vi "gyro-pll-V3.vi"() -> ()   [LabVIEW 2018]
uses:
  lorentzian.ctl
  circle corners.ctl
  pid -- parameters.ctl
  <vilib>/event_ctls.llb/eventvkey.ctl
  show-win- control.ctl
  server talk-to-back pair.ctl
  server talkback message type.ctl
  server talkto message type.ctl
  agregator -- action.ctl
  interpolation state - real.ctl
  pll internal user event action.ctl
  publisher action.ctl
  four-corner circle transformation.ctl
  cursor action.ctl
  Q -- check range -- i -- real.vi
  linear interpolation - real.vi
  draw a circle.vi
  linear interpolation iiii- complex.vi
  <vilib>/Analysis/baseanly.llb/A x B.vi
  <vilib>/Analysis/baseanly.llb/Complex A x B.vi
  line -- complex.vi
  Q -- check range -- i -- integer.vi
  generate linear region.vi
  Q - not nan -- real.vi
  Q - not nan -- integer.vi
  <vilib>/Analysis/Matrix/Numeric/Conversions/Array To Matrix.vi
  <vilib>/Analysis/Matrix/Numeric/Conversions/Array To Matrix - RA2.vi
  <vilib>/Analysis/baseanly.llb/Inverse Matrix.vi
  <vilib>/Analysis/baseanly.llb/Real Inverse Matrix.vi
panel:
  in  "(*) sweeper server":bool=TRUE
  in  "(*) pll":bool
  in  "exit!":bool
  in  "(*) sourcer":bool
  in  "(*) fitter":bool
  in  "(*) sweeper":bool=TRUE
  in  "all 3":T1(tab)
  in  "reset lor! :q":bool
  in  "Tab Control":enum32{"PID", "hist", "params"}(tab)=enum."params"
  in  "PID parameters :{}[];'":T2={"I (sec)"=0.004634123928756344, "P (sec)"=0.008980860327047186} {"P (sec)" scale=0.01..10.0; "I (sec)" scale=0.01..10.0}
  out "Plot: complex- hist":cluster{dbl[], dbl[]}[](graph)=[{array[1000 elements], array[1000 elements]}, {[7.190597353205284e-06, 7.172141018125027e-06, 7.116804391567491e-06, 7.024684552779172e-06, 6.895943111259833e-06, 6.7308059232445354e-06, 6.529562695475053e-06, 6.292566476955803e-06, 6.020233039585921e-06, 5.713040148754082e-06, 5.371526725175644e-06, 4.996291899442611e-06, 4.5879939609449636e-06, 4.147349203007406e-06, 3.6751306662674513e-06, 3.1721667824994774e-06, 2.6393399212638878e-06, 2.0775848419310813e-06, 1.4878870537958579e-06, 8.712810871592677e-07, 2.2884867841089993e-07, -4.382831277042918e-07, -1.1289439553054788e-06, -1.8419221506129192e-06, -2.575966907600425e-06, -3.329790462334158e-06, -4.102070352148148e-06, -4.891451735693187e-06, -5.696549769788949e-06, -6.515952038909475e-06, -7.348221033039968e-06, -8.191896669557811e-06, -9.045498854713654e-06, -9.907530080218758e-06, -1.0776478050383408e-05, -1.1650818335197432e-05, -1.252901704469844e-05, -1.3409533519936043e-05, -1.4290823035811157e-05, -1.5171339511048758e-05, -1.6049538220549768e-05, -1.692387850536379e-05, -1.7792826475528438e-05, -1.8654857701033543e-05, -1.950845988618939e-05, -2.035213552270723e-05, -2.1184404516837726e-05, -2.200380678595825e-05, -2.2808904820054008e-05, -2.3598286203599055e-05, -2.4370566093413044e-05, -2.5124389648146775e-05, -2.5858434405134282e-05, -2.6571412600441725e-05, -2.7262073428042906e-05, -2.79292052341581e-05, -2.8571637642906468e-05, -2.918824360954306e-05, -2.9777941397678286e-05, -3.0339696477011096e-05, -3.087252333824668e-05, -3.137548722201465e-05, -3.184770575875461e-05, -3.228835051669217e-05, -3.269664845518981e-05, -3.3071883280922845e-05, -3.341339670450129e-05, -3.372058959533313e-05, -3.399292303270301e-05, -3.4229919251222255e-05, -3.4431162478991744e-05, -3.4596299667007035e-05, -3.472504110852638e-05, -3.4817160947314696e-05, -3.4872497573872235e-05, -3.489095390895249e-05, -3.4872497573872235e-05, -3.4817160947314696e-05, -3.472504110852638e-05, -3.459629966700704e-05, -3.4431162478991744e-05, -3.422991925122226e-05, -3.3992923032703014e-05, -3.372058959533313e-05, -3.341339670450129e-05, -3.307188328092285e-05, -3.269664845518982e-05, -3.2288350516692175e-05, -3.1847705758754615e-05, -3.137548722201466e-05, -3.087252333824669e-05, -3.0339696477011103e-05, -2.9777941397678293e-05, -2.9188243609543066e-05, -2.8571637642906474e-05, -2.7929205234158112e-05, -2.726207342804292e-05, -2.6571412600441735e-05, -2.5858434405134296e-05, -2.512438964814679e-05, -2.4370566093413057e-05, -2.3598286203599066e-05, -2.280890482005402e-05, -2.200380678595826e-05, -2.1184404516837737e-05, -2.035213552270724e-05, -1.9508459886189396e-05, -1.865485770103357e-05, -1.7792826475528462e-05, -1.6923878505363813e-05, -1.6049538220549788e-05, -1.5171339511048779e-05, -1.4290823035811176e-05, -1.3409533519936056e-05, -1.2529017044698455e-05, -1.1650818335197446e-05, -1.0776478050383421e-05, -9.907530080218769e-06, -9.045498854713664e-06, -8.19189666955782e-06, -7.348221033039972e-06, -6.515952038909498e-06, -5.69654976978897e-06, -4.891451735693207e-06, -4.102070352148165e-06, -3.3297904623341733e-06, -2.575966907600442e-06, -1.8419221506129327e-06, -1.1289439553054907e-06, -4.3828312770430365e-07, 2.2884867841089146e-07, 8.712810871592576e-07, 1.4878870537958511e-06, 2.0775848419310745e-06, 2.6393399212638844e-06, 3.172166782499474e-06, 3.6751306662674378e-06, 4.147349203007396e-06, 4.587993960944957e-06, 4.996291899442601e-06, 5.371526725175637e-06, 5.713040148754075e-06, 6.020233039585914e-06, 6.292566476955799e-06, 6.52956269547505e-06, 6.7308059232445354e-06, 6.89594311125983e-06, 7.024684552779168e-06, 7.116804391567491e-06, 7.172141018125027e-06], [0.0002113633008955132, 0.00021224439713003404, 0.00021312394762236102, 0.00021400040934205735, 0.00021487224467744295, 0.00021573792413308792, 0.00021659592901306725, 0.0002174447540852694, 0.00021828291022208502, 0.0002191089270128428, 0.00021992135534340933, 0.00022071876993842783, 0.00022149977186173528, 0.00022226299097057205, 0.00022300708831927754, 0.00022373075850825623, 0.00022443273197409182, 0.00022511177721679307, 0.00022576670296026313, 0.00022639636024220273, 0.00022699964442978034, 0.0002275754971575336, 0.000228122908184102, 0.00022864091716453335, 0.0002291286153350554, 0.0002295851471073561, 0.00023000971156957625, 0.00023040156389138116, 0.0002307600166306461, 0.00023108444093946333, 0.00023137426766735506, 0.00023162898835975677, 0.0002318481561500193, 0.00023203138654336486, 0.0002321783580914214, 0.00023228881295615236, 0.00023236255736219216, 0.00023239946193679412, 0.00023239946193679412, 0.00023236255736219216, 0.00023228881295615236, 0.0002321783580914214, 0.00023203138654336486, 0.0002318481561500193, 0.00023162898835975677, 0.00023137426766735506, 0.00023108444093946333, 0.00023076001663064613, 0.00023040156389138116, 0.00023000971156957625, 0.0002295851471073561, 0.0002291286153350554, 0.00022864091716453335, 0.000228122908184102, 0.0002275754971575336, 0.00022699964442978034, 0.00022639636024220273, 0.00022576670296026315, 0.00022511177721679307, 0.00022443273197409182, 0.00022373075850825623, 0.00022300708831927757, 0.00022226299097057205, 0.0002214997718617353, 0.00022071876993842783, 0.00021992135534340933, 0.0002191089270128428, 0.00021828291022208502, 0.0002174447540852694, 0.00021659592901306725, 0.00021573792413308792, 0.00021487224467744295, 0.00021400040934205735, 0.00021312394762236102, 0.00021224439713003404, 0.0002113633008955132, 0.00021048220466099237, 0.0002096026541686654, 0.0002087261924489691, 0.0002078543571135835, 0.0002069886776579385, 0.00020613067277795916, 0.00020528184770575705, 0.00020444369156894142, 0.00020361767477818362, 0.00020280524644761708, 0.0002020078318525986, 0.00020122682992929113, 0.0002004636108204544, 0.00019971951347174887, 0.00019899584328277018, 0.0001982938698169346, 0.00019761482457423337, 0.0001969598988307633, 0.00019633024154882368, 0.00019572695736124607, 0.0001951511046334928, 0.00019460369360692445, 0.00019408568462649307, 0.00019359798645597102, 0.00019314145468367035, 0.0001927168902214502, 0.00019232503789964525, 0.0001919665851603803, 0.00019164216085156309, 0.00019135233412367135, 0.00019109761343126964, 0.0001908784456410071, 0.00019069521524766155, 0.000190548243699605, 0.00019043778883487406, 0.00019036404442883425, 0.0001903271398542323, 0.0001903271398542323, 0.00019036404442883425, 0.00019043778883487406, 0.000190548243699605, 0.00019069521524766155, 0.0001908784456410071, 0.00019109761343126964, 0.00019135233412367135, 0.00019164216085156306, 0.00019196658516038029, 0.00019232503789964523, 0.00019271689022145016, 0.00019314145468367033, 0.000193597986455971, 0.00019408568462649307, 0.00019460369360692443, 0.0001951511046334928, 0.00019572695736124607, 0.00019633024154882368, 0.00019695989883076326, 0.00019761482457423334, 0.0001982938698169346, 0.00019899584328277018, 0.00019971951347174885, 0.00020046361082045436, 0.0002012268299292911, 0.00020200783185259858, 0.00020280524644761705, 0.0002036176747781836, 0.0002044436915689414, 0.00020528184770575702, 0.00020613067277795916, 0.0002069886776579385, 0.00020785435711358346, 0.00020872619244896907, 0.00020960265416866537, 0.00021048220466099237]}, {[7.168586400274939e-06, 5.066709932460086e-06, 2.964833464645231e-06, 8.629569968303764e-07, -1.2389194709844774e-06, -3.340795938799331e-06, -5.442672406614187e-06, -7.54454887442904e-06, -9.646425342243894e-06, -1.174830181005875e-05, -1.3850178277873602e-05, -1.5952054745688457e-05, -1.8053931213503313e-05, -2.0155807681318165e-05, -2.225768414913302e-05, -2.4359560616947872e-05, -2.6461437084762728e-05, -2.8563313552577583e-05, -3.066519002039244e-05, -3.276706648820729e-05], [0.00021232547061132137, 0.00021222925363974056, 0.00021213303666815973, 0.00021203681969657892, 0.0002119406027249981, 0.0002118443857534173, 0.00021174816878183648, 0.00021165195181025565, 0.00021155573483867484, 0.000211459517867094, 0.0002113633008955132, 0.0002112670839239324, 0.00021117086695235157, 0.00021107464998077076, 0.00021097843300918993, 0.00021088221603760913, 0.00021078599906602832, 0.0002106897820944475, 0.00021059356512286668, 0.00021049734815128585]}, {[-1.288800856206544e-05, -1.2984225533646258e-05, -1.3080442505227073e-05, -1.317665947680789e-05, -1.3272876448388706e-05, -1.3369093419969523e-05, -1.3465310391550338e-05, -1.3561527363131155e-05, -1.365774433471197e-05, -1.3753961306292788e-05, -1.3850178277873605e-05, -1.394639524945442e-05, -1.4042612221035236e-05, -1.4138829192616053e-05, -1.423504616419687e-05, -1.4331263135777686e-05, -1.4427480107358503e-05, -1.4523697078939318e-05, -1.4619914050520135e-05, -1.471613102210095e-05], [0.00019034453621736468, 0.00019244641268517952, 0.0001945482891529944, 0.00019665016562080923, 0.0001987520420886241, 0.00020085391855643894, 0.00020295579502425378, 0.00020505767149206865, 0.0002071595479598835, 0.00020926142442769836, 0.0002113633008955132, 0.00021346517736332805, 0.00021556705383114292, 0.00021766893029895776, 0.00021977080676677263, 0.00022187268323458747, 0.0002239745597024023, 0.00022607643617021718, 0.00022817831263803202, 0.0002302801891058469]}, {[9.092925831891258e-06, 8.900491888729626e-06, 8.708057945567993e-06, 8.515624002406362e-06, 8.32319005924473e-06, 8.130756116083097e-06, 7.938322172921465e-06, 7.745888229759832e-06, 7.5534542865982e-06, 7.361020343436568e-06, 7.168586400274936e-06, 6.976152457113303e-06, 6.783718513951671e-06, 6.591284570790038e-06, 6.3988506276284065e-06, 6.206416684466774e-06, 6.013982741305142e-06, 5.82154879814351e-06, 5.629114854981877e-06, 5.4366809118202445e-06], [0.0001702879412550243, 0.00017449169419065402, 0.00017869544712628373, 0.00018289920006191342, 0.00018710295299754313, 0.00019130670593317284, 0.00019551045886880255, 0.00019971421180443226, 0.00020391796474006197, 0.00020812171767569168, 0.00021232547061132137, 0.00021652922354695108, 0.0002207329764825808, 0.0002249367294182105, 0.0002291404823538402, 0.0002333442352894699, 0.00023754798822509963, 0.00024175174116072932, 0.00024595549409635905, 0.00025015924703198874]}, {[-1.97103396318906e-05, -1.91243234964889e-05, -1.8538307361087202e-05, -1.79522912256855e-05, -1.73662750902838e-05, -1.6780258954882103e-05, -1.6194242819480402e-05, -1.5608226684078704e-05, -1.5022210548677003e-05, -1.4436194413275303e-05, -1.3850178277873603e-05, -1.3264162142471904e-05, -1.2678146007070203e-05, -1.2092129871668504e-05, -1.1506113736266805e-05, -1.0920097600865104e-05, -1.0334081465463405e-05, -9.748065330061706e-06, -9.162049194660005e-06, -8.576033059258306e-06], [0.00023375398508080204, 0.00023151491666227315, 0.00022927584824374426, 0.0002270367798252154, 0.0002247977114066865, 0.00022255864298815762, 0.00022031957456962873, 0.00021808050615109985, 0.00021584143773257098, 0.0002136023693140421, 0.0002113633008955132, 0.00020912423247698432, 0.00020688516405845543, 0.00020464609563992657, 0.00020240702722139768, 0.0002001679588028688, 0.0001979288903843399, 0.00019568982196581104, 0.00019345075354728215, 0.00019121168512875326]}]
  in  "dt (sec)":dbl=0.001 format="%#_10f"
  in  "plot hist time (sec)":dbl=1.0 format="%#_10f"
  out "G (Hz)":dbl=6.817921124952451 format="%#.4f"
  in  "reset freq! :r":bool
  out "Plot: complex plane":cluster{dbl[], dbl[]}[](graph)=[{[7.190597353205284e-06, 7.172141018125027e-06, 7.116804391567491e-06, 7.024684552779172e-06, 6.895943111259833e-06, 6.7308059232445354e-06, 6.529562695475053e-06, 6.292566476955803e-06, 6.020233039585921e-06, 5.713040148754082e-06, 5.371526725175644e-06, 4.996291899442611e-06, 4.5879939609449636e-06, 4.147349203007406e-06, 3.6751306662674513e-06, 3.1721667824994774e-06, 2.6393399212638878e-06, 2.0775848419310813e-06, 1.4878870537958579e-06, 8.712810871592677e-07, 2.2884867841089993e-07, -4.382831277042918e-07, -1.1289439553054788e-06, -1.8419221506129192e-06, -2.575966907600425e-06, -3.329790462334158e-06, -4.102070352148148e-06, -4.891451735693187e-06, -5.696549769788949e-06, -6.515952038909475e-06, -7.348221033039968e-06, -8.191896669557811e-06, -9.045498854713654e-06, -9.907530080218758e-06, -1.0776478050383408e-05, -1.1650818335197432e-05, -1.252901704469844e-05, -1.3409533519936043e-05, -1.4290823035811157e-05, -1.5171339511048758e-05, -1.6049538220549768e-05, -1.692387850536379e-05, -1.7792826475528438e-05, -1.8654857701033543e-05, -1.950845988618939e-05, -2.035213552270723e-05, -2.1184404516837726e-05, -2.200380678595825e-05, -2.2808904820054008e-05, -2.3598286203599055e-05, -2.4370566093413044e-05, -2.5124389648146775e-05, -2.5858434405134282e-05, -2.6571412600441725e-05, -2.7262073428042906e-05, -2.79292052341581e-05, -2.8571637642906468e-05, -2.918824360954306e-05, -2.9777941397678286e-05, -3.0339696477011096e-05, -3.087252333824668e-05, -3.137548722201465e-05, -3.184770575875461e-05, -3.228835051669217e-05, -3.269664845518981e-05, -3.3071883280922845e-05, -3.341339670450129e-05, -3.372058959533313e-05, -3.399292303270301e-05, -3.4229919251222255e-05, -3.4431162478991744e-05, -3.4596299667007035e-05, -3.472504110852638e-05, -3.4817160947314696e-05, -3.4872497573872235e-05, -3.489095390895249e-05, -3.4872497573872235e-05, -3.4817160947314696e-05, -3.472504110852638e-05, -3.459629966700704e-05, -3.4431162478991744e-05, -3.422991925122226e-05, -3.3992923032703014e-05, -3.372058959533313e-05, -3.341339670450129e-05, -3.307188328092285e-05, -3.269664845518982e-05, -3.2288350516692175e-05, -3.1847705758754615e-05, -3.137548722201466e-05, -3.087252333824669e-05, -3.0339696477011103e-05, -2.9777941397678293e-05, -2.9188243609543066e-05, -2.8571637642906474e-05, -2.7929205234158112e-05, -2.726207342804292e-05, -2.6571412600441735e-05, -2.5858434405134296e-05, -2.512438964814679e-05, -2.4370566093413057e-05, -2.3598286203599066e-05, -2.280890482005402e-05, -2.200380678595826e-05, -2.1184404516837737e-05, -2.035213552270724e-05, -1.9508459886189396e-05, -1.865485770103357e-05, -1.7792826475528462e-05, -1.6923878505363813e-05, -1.6049538220549788e-05, -1.5171339511048779e-05, -1.4290823035811176e-05, -1.3409533519936056e-05, -1.2529017044698455e-05, -1.1650818335197446e-05, -1.0776478050383421e-05, -9.907530080218769e-06, -9.045498854713664e-06, -8.19189666955782e-06, -7.348221033039972e-06, -6.515952038909498e-06, -5.69654976978897e-06, -4.891451735693207e-06, -4.102070352148165e-06, -3.3297904623341733e-06, -2.575966907600442e-06, -1.8419221506129327e-06, -1.1289439553054907e-06, -4.3828312770430365e-07, 2.2884867841089146e-07, 8.712810871592576e-07, 1.4878870537958511e-06, 2.0775848419310745e-06, 2.6393399212638844e-06, 3.172166782499474e-06, 3.6751306662674378e-06, 4.147349203007396e-06, 4.587993960944957e-06, 4.996291899442601e-06, 5.371526725175637e-06, 5.713040148754075e-06, 6.020233039585914e-06, 6.292566476955799e-06, 6.52956269547505e-06, 6.7308059232445354e-06, 6.89594311125983e-06, 7.024684552779168e-06, 7.116804391567491e-06, 7.172141018125027e-06], [0.0002113633008955132, 0.00021224439713003404, 0.00021312394762236102, 0.00021400040934205735, 0.00021487224467744295, 0.00021573792413308792, 0.00021659592901306725, 0.0002174447540852694, 0.00021828291022208502, 0.0002191089270128428, 0.00021992135534340933, 0.00022071876993842783, 0.00022149977186173528, 0.00022226299097057205, 0.00022300708831927754, 0.00022373075850825623, 0.00022443273197409182, 0.00022511177721679307, 0.00022576670296026313, 0.00022639636024220273, 0.00022699964442978034, 0.0002275754971575336, 0.000228122908184102, 0.00022864091716453335, 0.0002291286153350554, 0.0002295851471073561, 0.00023000971156957625, 0.00023040156389138116, 0.0002307600166306461, 0.00023108444093946333, 0.00023137426766735506, 0.00023162898835975677, 0.0002318481561500193, 0.00023203138654336486, 0.0002321783580914214, 0.00023228881295615236, 0.00023236255736219216, 0.00023239946193679412, 0.00023239946193679412, 0.00023236255736219216, 0.00023228881295615236, 0.0002321783580914214, 0.00023203138654336486, 0.0002318481561500193, 0.00023162898835975677, 0.00023137426766735506, 0.00023108444093946333, 0.00023076001663064613, 0.00023040156389138116, 0.00023000971156957625, 0.0002295851471073561, 0.0002291286153350554, 0.00022864091716453335, 0.000228122908184102, 0.0002275754971575336, 0.00022699964442978034, 0.00022639636024220273, 0.00022576670296026315, 0.00022511177721679307, 0.00022443273197409182, 0.00022373075850825623, 0.00022300708831927757, 0.00022226299097057205, 0.0002214997718617353, 0.00022071876993842783, 0.00021992135534340933, 0.0002191089270128428, 0.00021828291022208502, 0.0002174447540852694, 0.00021659592901306725, 0.00021573792413308792, 0.00021487224467744295, 0.00021400040934205735, 0.00021312394762236102, 0.00021224439713003404, 0.0002113633008955132, 0.00021048220466099237, 0.0002096026541686654, 0.0002087261924489691, 0.0002078543571135835, 0.0002069886776579385, 0.00020613067277795916, 0.00020528184770575705, 0.00020444369156894142, 0.00020361767477818362, 0.00020280524644761708, 0.0002020078318525986, 0.00020122682992929113, 0.0002004636108204544, 0.00019971951347174887, 0.00019899584328277018, 0.0001982938698169346, 0.00019761482457423337, 0.0001969598988307633, 0.00019633024154882368, 0.00019572695736124607, 0.0001951511046334928, 0.00019460369360692445, 0.00019408568462649307, 0.00019359798645597102, 0.00019314145468367035, 0.0001927168902214502, 0.00019232503789964525, 0.0001919665851603803, 0.00019164216085156309, 0.00019135233412367135, 0.00019109761343126964, 0.0001908784456410071, 0.00019069521524766155, 0.000190548243699605, 0.00019043778883487406, 0.00019036404442883425, 0.0001903271398542323, 0.0001903271398542323, 0.00019036404442883425, 0.00019043778883487406, 0.000190548243699605, 0.00019069521524766155, 0.0001908784456410071, 0.00019109761343126964, 0.00019135233412367135, 0.00019164216085156306, 0.00019196658516038029, 0.00019232503789964523, 0.00019271689022145016, 0.00019314145468367033, 0.000193597986455971, 0.00019408568462649307, 0.00019460369360692443, 0.0001951511046334928, 0.00019572695736124607, 0.00019633024154882368, 0.00019695989883076326, 0.00019761482457423334, 0.0001982938698169346, 0.00019899584328277018, 0.00019971951347174885, 0.00020046361082045436, 0.0002012268299292911, 0.00020200783185259858, 0.00020280524644761705, 0.0002036176747781836, 0.0002044436915689414, 0.00020528184770575702, 0.00020613067277795916, 0.0002069886776579385, 0.00020785435711358346, 0.00020872619244896907, 0.00020960265416866537, 0.00021048220466099237]}, {[7.168586400274939e-06, 5.066709932460086e-06, 2.964833464645231e-06, 8.629569968303764e-07, -1.2389194709844774e-06, -3.340795938799331e-06, -5.442672406614187e-06, -7.54454887442904e-06, -9.646425342243894e-06, -1.174830181005875e-05, -1.3850178277873602e-05, -1.5952054745688457e-05, -1.8053931213503313e-05, -2.0155807681318165e-05, -2.225768414913302e-05, -2.4359560616947872e-05, -2.6461437084762728e-05, -2.8563313552577583e-05, -3.066519002039244e-05, -3.276706648820729e-05], [0.00021232547061132137, 0.00021222925363974056, 0.00021213303666815973, 0.00021203681969657892, 0.0002119406027249981, 0.0002118443857534173, 0.00021174816878183648, 0.00021165195181025565, 0.00021155573483867484, 0.000211459517867094, 0.0002113633008955132, 0.0002112670839239324, 0.00021117086695235157, 0.00021107464998077076, 0.00021097843300918993, 0.00021088221603760913, 0.00021078599906602832, 0.0002106897820944475, 0.00021059356512286668, 0.00021049734815128585]}, {[-1.288800856206544e-05, -1.2984225533646258e-05, -1.3080442505227073e-05, -1.317665947680789e-05, -1.3272876448388706e-05, -1.3369093419969523e-05, -1.3465310391550338e-05, -1.3561527363131155e-05, -1.365774433471197e-05, -1.3753961306292788e-05, -1.3850178277873605e-05, -1.394639524945442e-05, -1.4042612221035236e-05, -1.4138829192616053e-05, -1.423504616419687e-05, -1.4331263135777686e-05, -1.4427480107358503e-05, -1.4523697078939318e-05, -1.4619914050520135e-05, -1.471613102210095e-05], [0.00019034453621736468, 0.00019244641268517952, 0.0001945482891529944, 0.00019665016562080923, 0.0001987520420886241, 0.00020085391855643894, 0.00020295579502425378, 0.00020505767149206865, 0.0002071595479598835, 0.00020926142442769836, 0.0002113633008955132, 0.00021346517736332805, 0.00021556705383114292, 0.00021766893029895776, 0.00021977080676677263, 0.00022187268323458747, 0.0002239745597024023, 0.00022607643617021718, 0.00022817831263803202, 0.0002302801891058469]}, {[9.092925831891258e-06, 8.900491888729626e-06, 8.708057945567993e-06, 8.515624002406362e-06, 8.32319005924473e-06, 8.130756116083097e-06, 7.938322172921465e-06, 7.745888229759832e-06, 7.5534542865982e-06, 7.361020343436568e-06, 7.168586400274936e-06, 6.976152457113303e-06, 6.783718513951671e-06, 6.591284570790038e-06, 6.3988506276284065e-06, 6.206416684466774e-06, 6.013982741305142e-06, 5.82154879814351e-06, 5.629114854981877e-06, 5.4366809118202445e-06], [0.0001702879412550243, 0.00017449169419065402, 0.00017869544712628373, 0.00018289920006191342, 0.00018710295299754313, 0.00019130670593317284, 0.00019551045886880255, 0.00019971421180443226, 0.00020391796474006197, 0.00020812171767569168, 0.00021232547061132137, 0.00021652922354695108, 0.0002207329764825808, 0.0002249367294182105, 0.0002291404823538402, 0.0002333442352894699, 0.00023754798822509963, 0.00024175174116072932, 0.00024595549409635905, 0.00025015924703198874]}]
  in  "lorentzian":T3={"A (VHz)"=0.0007250653088846297, "f (Hz)"=45017.43809779818, "G (Hz)"=34.46000858512321, "phi(rad)"=-1.525051560312372, "Q"=1306.3675821959234, "Norm  Ampl"=nan, "bg (V)"=7.168586400274938e-06+0.00021232547061132137i, "4corners"={"z (-pi/2)"=-1.288800856206544e-05+0.00019034453621736468i, "z(inf)"=7.168586400274938e-06+0.00021232547061132137i, "z (pi/2)"=-1.4812347993681768e-05+0.00023238206557366173i, "z center"=-1.3850178277873603e-05+0.0002113633008955132i, "z(0)"=-3.486894295602214e-05+0.00021040113117970505i, "radius"=2.1040775631078887e-05}} {"bg (V)" format="%#9_9f"; "Q" format="%#9_9f"; "phi(rad)" format="%#9_9f"; "G (Hz)" format="%#9_9f"; "f (Hz)" format="%#9_9f"}
  in  "toggle PLL! :@":bool
  out "f (Hz)":dbl=40017.438097734725 format="%#.11f"
  in  "PLL is ON":bool
  out "VKey":T5
  out "Char":i16=62
  in  "lorentzian -- basic":T3={"A (VHz)"=1.0, "f (Hz)"=1000.0, "G (Hz)"=3.0, "phi(rad)"=0.0, "Q"=300.0, "Norm  Ampl"=nan, "bg (V)"=0.0+0.0i, "4corners"={"z (-pi/2)"=9.277908004825974e-07+0.0007240755403629966i, "z(inf)"=2.6527949823343002e-05+0.0007477540585896028i, "z (pi/2)"=2.8494315967368497e-06+0.0007733542176124632i, "z center"=1.8886111986097237e-06+0.0007487148789877299i, "z(0)"=-2.2750727426123552e-05+0.000749675699385857i, "radius"=2.4658065287076567e-05}} {"bg (V)" format="%#9_9f"; "Q" format="%#9_9f"; "phi(rad)" format="%#9_9f"; "G (Hz)" format="%#9_9f"; "f (Hz)" format="%#9_9f"}
  in  "save lor for later":bool
  in  "reset lorentzian from basic":bool
  out "zi out Im (V)":dbl=-2.55535250615244e-07 format="%#.8f"
  out "zi out Re (V)":dbl=2.3785838016890924e-07 format="%#.8f"
  out "publish message":T6
  out "Stoped?":bool
  out "window":T7={"cen (Hz)"=45496.74569300777, "win (Hz)"=29.962105514646385, "left (Hz)"=45481.76464025045, "right (Hz)"=45511.72674576509}
  in  "lorentzian -- hist":T3={"A (VHz)"=0.0007250653088846297, "f (Hz)"=45017.43809779818, "G (Hz)"=34.46000858512321, "phi(rad)"=-1.525051560312372, "Q"=1306.3675821959234, "Norm  Ampl"=nan, "bg (V)"=7.168586400274938e-06+0.00021232547061132137i, "4corners"={"z (-pi/2)"=-1.288800856206544e-05+0.00019034453621736468i, "z(inf)"=7.168586400274938e-06+0.00021232547061132137i, "z (pi/2)"=-1.4812347993681768e-05+0.00023238206557366173i, "z center"=-1.3850178277873603e-05+0.0002113633008955132i, "z(0)"=-3.486894295602214e-05+0.00021040113117970505i, "radius"=2.1040775631078887e-05}} {"bg (V)" format="%#9_9f"; "Q" format="%#9_9f"; "phi(rad)" format="%#9_9f"; "G (Hz)" format="%#9_9f"; "f (Hz)" format="%#9_9f"}
  out "pll event pair":T8
  out "sweeper server reference":refnum<vi>
  out "pll async reference":refnum<vi>
  out "async fitter":refnum<vi>
  out "async sweeper":refnum<vi>
  out "fitter event pair":T8
  out "sweeper event pair":T8
  out "async sourcer":refnum<vi>
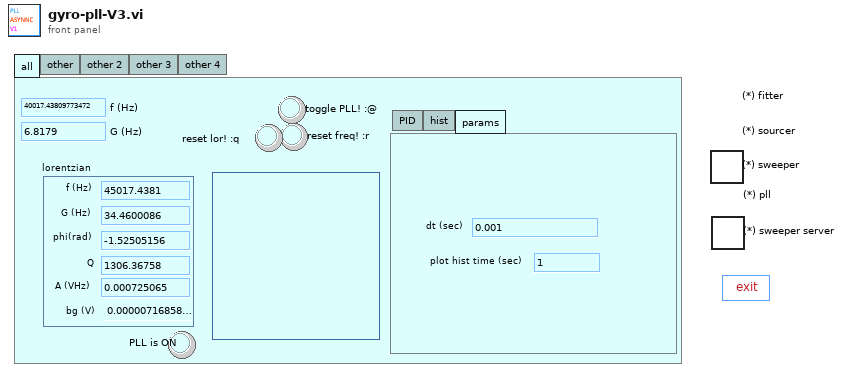
[diagram p1: front panel]
types:
  T1 = enum32{"all", "other", "other 2", "other 3", "other 4"}
  T2 = typedef "pid -- parameters.ctl" = cluster{"I (sec)":dbl, "P (sec)":dbl}
  T3 = typedef "lorentzian.ctl" = cluster{"A (VHz)":dbl, "f (Hz)":dbl, "G (Hz)":dbl, "phi(rad)":dbl, "Q":dbl, "Norm  Ampl":dbl, "bg (V)":cdb, "4corners":T4}
  T4 = typedef "circle corners.ctl" = cluster{"z (-pi/2)":cdb, "z(inf)":cdb, "z (pi/2)":cdb, "z center":cdb, "z(0)":cdb, "radius":dbl}
  T5 = typedef "eventvkey.ctl" = enum16{"ASCII", "Enter", "Return", "Shift", "Ctrl", "Alt", "Cmd", "Opt", "Caps", "NumLock", "Clear", "Break", "Up", "Down", "Left", "Right", "Insert", "Delete", "Home", "End", "PageUp", "PageDown", "Escape", "Help", "Pause", "ScrollLock", "F1", "F2", "F3", "F4", "F5", "F6", "F7", "F8", "F9", "F10", "F11", "F12", "F13", "F14", "F15", "F16", "F17", "F18", "F19", "F20", "F21", "F22", "F23", "F24", "Play", "VolumeUp", "VolumeDown", "Mute", "Two Byte Char"}
  T6 = cluster{"freq (Hz)":dbl, "gamma (Hz)":dbl, "Voltage (V)":cdb}
  T7 = typedef "show-win- control.ctl" = cluster{"cen (Hz)":dbl, "win (Hz)":dbl, "left (Hz)":dbl, "right (Hz)":dbl}
  T8 = typedef "server talk-to-back pair.ctl" = cluster{"talkback event":refnum<user-event>, "talkto event":refnum<user-event>}
  T9 = typedef "server talkback message type.ctl" = cluster{"message":enum16{"new", "void"}}
  T10 = typedef "server talkto message type.ctl" = cluster{"message":enum16{"stop", "start", "update pars", "update request", "new", "launch", "exit", "get", "reset", "pause", "unpause"}}
  T11 = typedef "pll internal user event action.ctl" = enum16{"gear pll async", "start pll async", "stop pll async", "toggle pll async", "gear sweeper", "start sweeper", "stop sweeper", "toggle sweeper", "accept frequency", "reset lorentzian", "accept lorentzian", "update cursors", "pause pll", "unpause pll", "void", "exit", "gear server sweeper", "gear sweeper async", "gear fitter", "gear sourcer"}
  T12 = typedef "interpolation state - real.ctl" = cluster{"requested size":i32, "Array":dbl[], "actual number of elements":i32}
  T13 = typedef "agregator -- action.ctl" = enum16{"append", "interpolate", "empty!", "force", "init", "scale", "read last"}
  T14 = typedef "publisher action.ctl" = enum16{"set", "get", "init", "check"}
  T15 = typedef "cursor action.ctl" = enum16{"range", "read", "write", "check", "zoom out", "smart zoom out", "zoom to aspect ratio 1", "zoom to win", "zoom out 20%", "zoom in 20%", "-empty", "smart zoom out&aspect", "move range left 20%", "move range right 20%", "move range up 20%", "move range down 20%", "zoom to X win", "zoom to Y win", "zoom out X", "zoom out Y", "zoom in X", "zoom in Y", "check plot scale"}
  T16 = typedef "four-corner circle transformation.ctl" = enum16{"z(c) z(inf)", "z(c) z(zero)", "fix phase", "calculate lorentzian", "z(0) z(+-pi/2)", "shift to zcenter", "to  canonical", "get canonical phase", "get4corners", "update lorentzian -- from z0", "fake gamma normal", "fake gamma heat", "calculate complex slope"}
  T17 = typedef "pll talkback data type.ctl" = cluster{"freq (Hz)":dbl, "gamma (Hz)":dbl, "Voltage (V)":cdb, "overlimit ?":bool}
  T18 = typedef "interpolation state - complex.ctl" = cluster{"requested size":i32, "Array":cdb[], "actual number of elements":i32}
  T19 = enum32{"Invalid", "Standard", "Closed", "Hidden", "Minimized", "Maximized"}
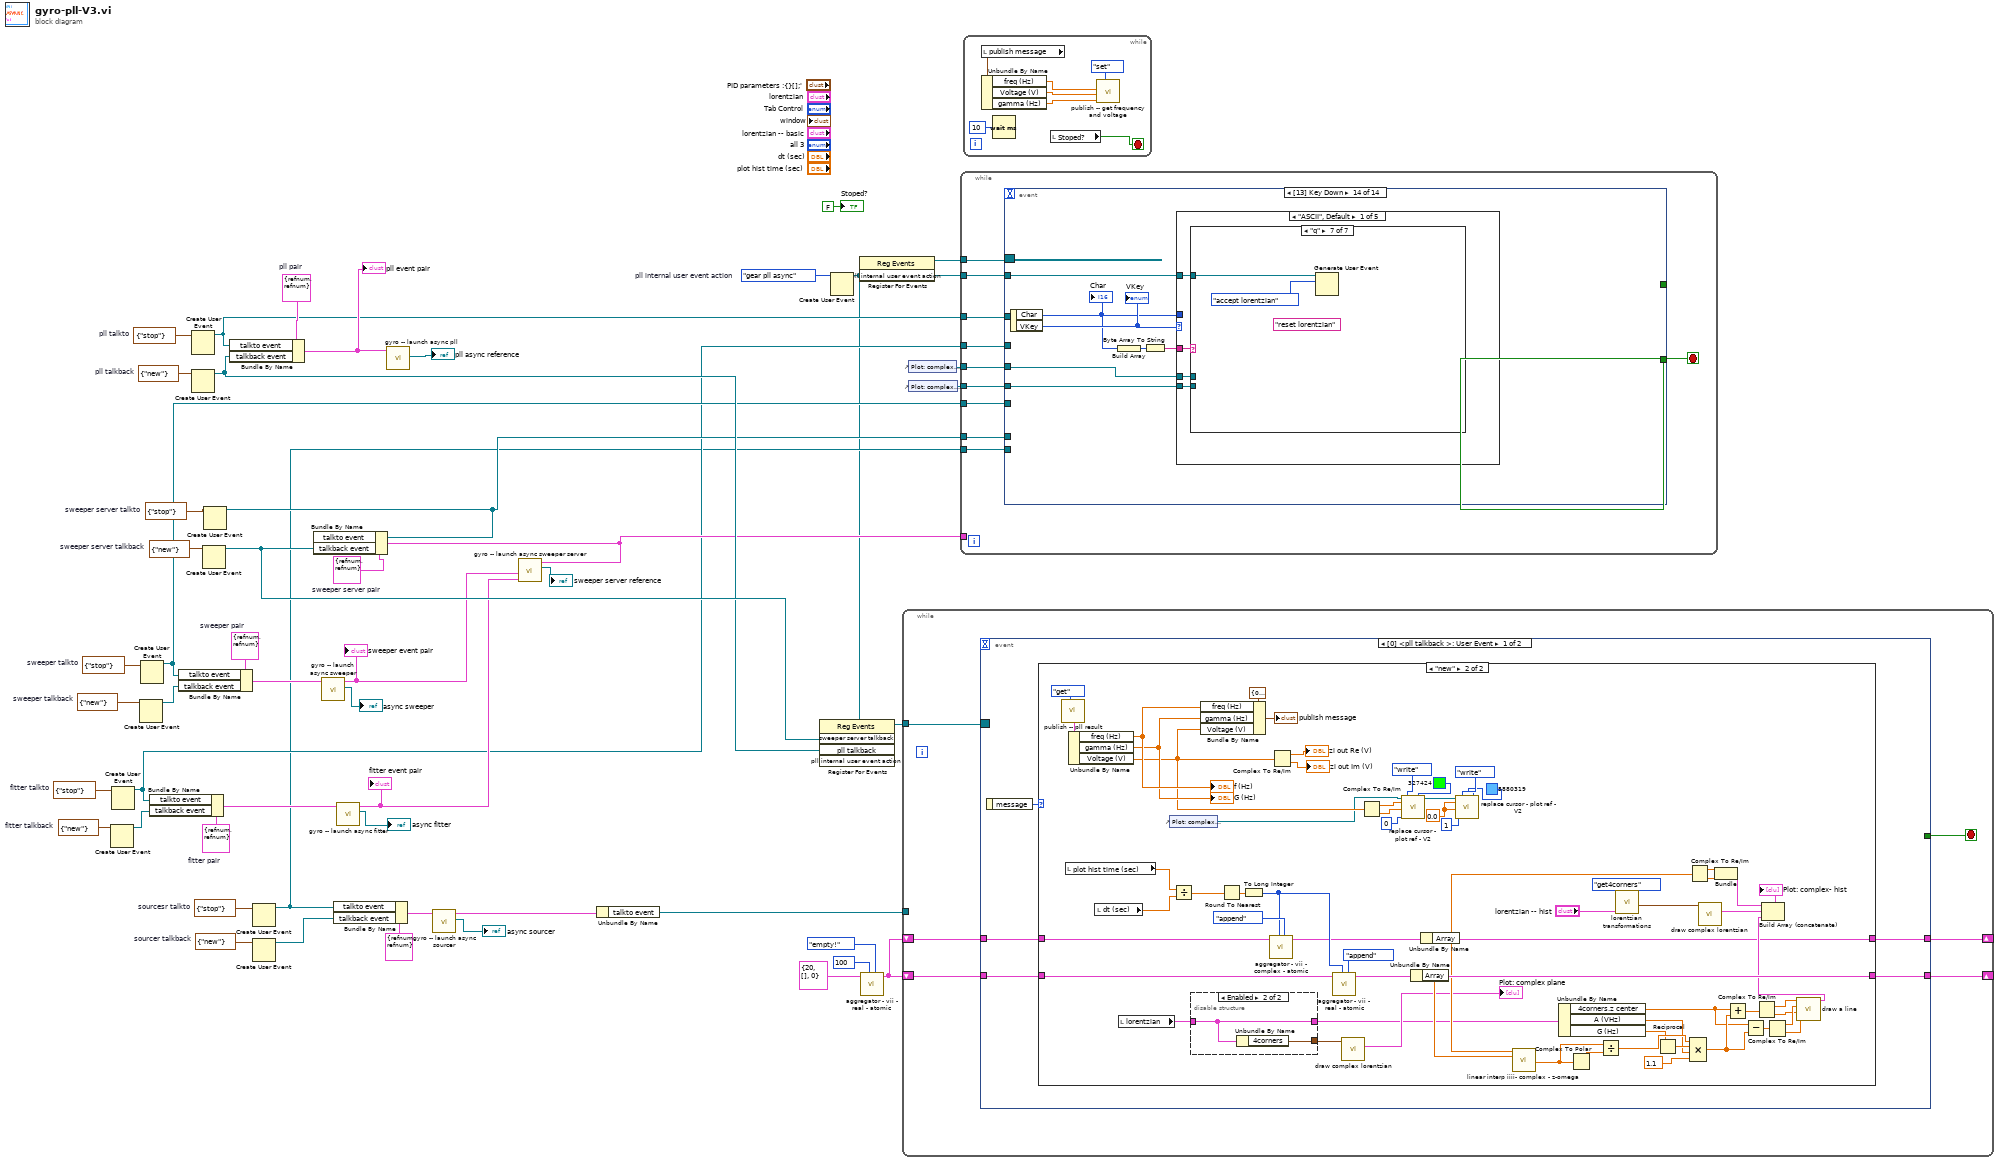
[diagram p0: block diagram]
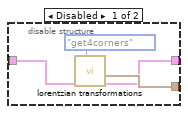
[diagram p3: hidden frame]
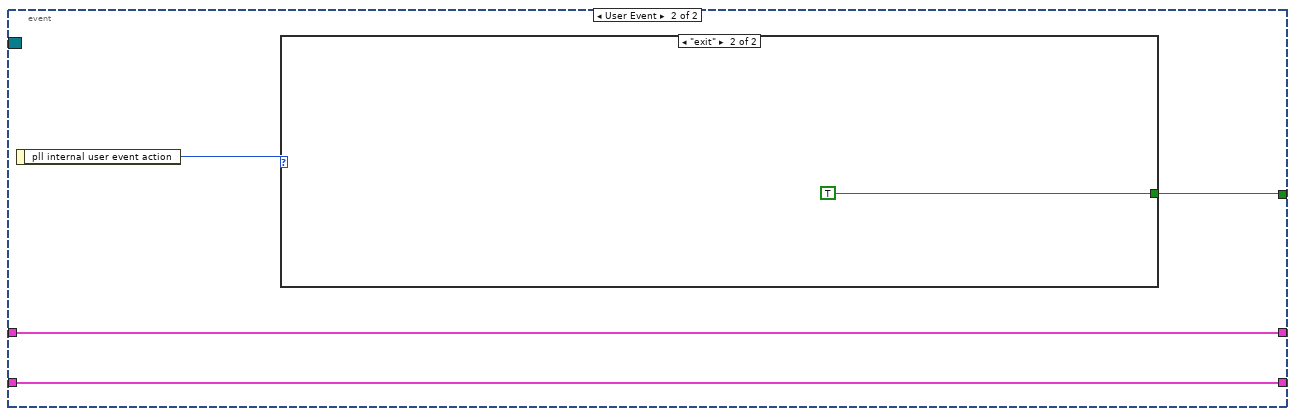
[diagram p4: hidden frame]
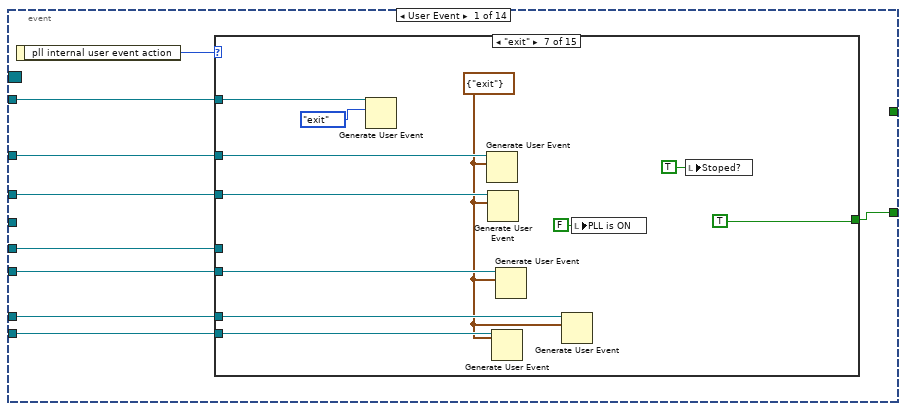
[diagram p6: hidden frame]
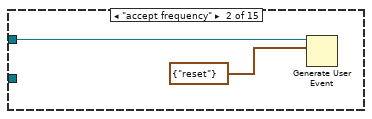
[diagram p8: hidden frame]
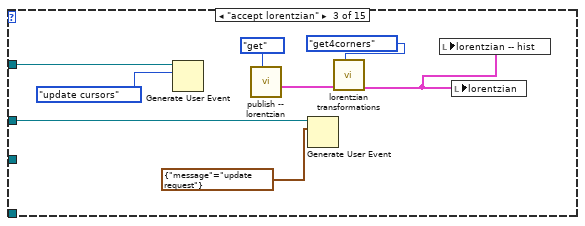
[diagram p9: hidden frame]
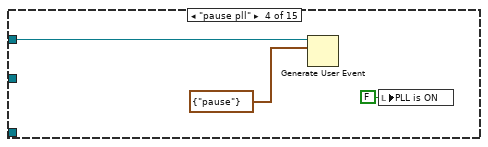
[diagram p10: hidden frame]
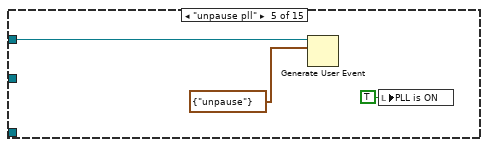
[diagram p11: hidden frame]
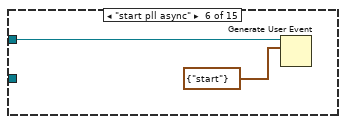
[diagram p12: hidden frame]
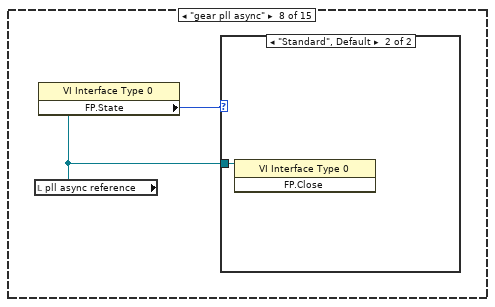
[diagram p13: hidden frame]
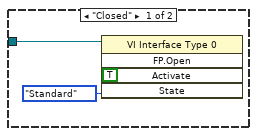
[diagram p14: hidden frame]
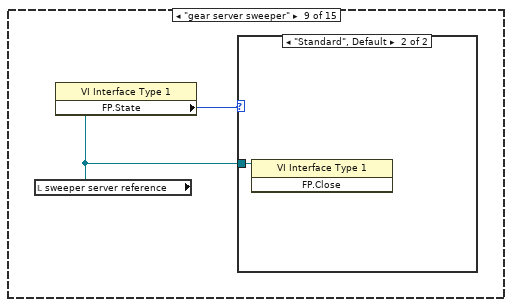
[diagram p15: hidden frame]
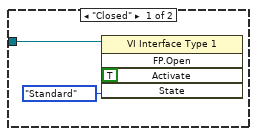
[diagram p16: hidden frame]
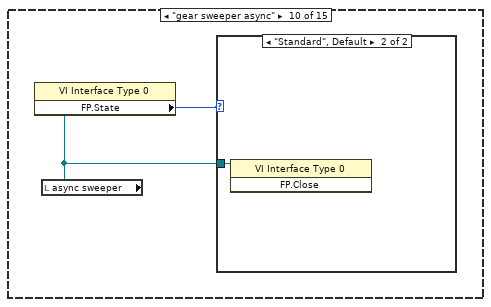
[diagram p17: hidden frame]
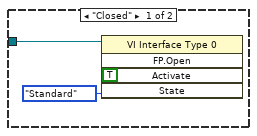
[diagram p18: hidden frame]
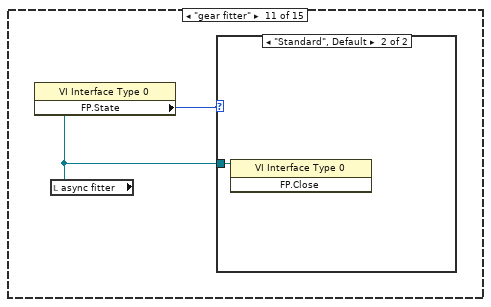
[diagram p19: hidden frame]
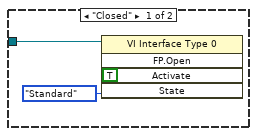
[diagram p20: hidden frame]
diagram:
  w11 = T9 {"message"=enum."new"}  # sourcer talkback
  w12 = T10 {"message"=enum."stop"}  # sourcesr talkto
  w22 = T8 {"talkback event"=refnum, "talkto event"=refnum}  # pll pair
  w20 = T9 {"message"=enum."new"}  # pll talkback
  w21 = T10 {"message"=enum."stop"}  # pll talkto
  w29 = T8 {"talkback event"=refnum, "talkto event"=refnum}  # sweeper server pair
  w27 = T9 {"message"=enum."new"}  # sweeper server talkback
  w28 = T10 {"message"=enum."stop"}  # sweeper server talkto
  w38 = T8 {"talkback event"=refnum, "talkto event"=refnum}  # sweeper pair
  w34 = T9 {"message"=enum."new"}  # sweeper talkback
  w35 = T10 {"message"=enum."stop"}  # sweeper talkto
  w39 = T8 {"talkback event"=refnum, "talkto event"=refnum}  # fitter pair
  w32 = T9 {"message"=enum."new"}  # fitter talkback
  w33 = T10 {"message"=enum."stop"}  # fitter talkto
  w42 = pll_internal_user_event_action."gear pll async"  # pll internal user event action
  n1 = Create User Event(user event datatype=w32) -> (user event=w25:refnum<user-event>)  [unwired: 1 in, 1 out]
  n2 = Create User Event(user event datatype=w33) -> (user event=w4:refnum<user-event>)  [unwired: 1 in, 1 out]
  n3 = Create User Event(user event datatype=w34) -> (user event=w30:refnum<user-event>)  [unwired: 1 in, 1 out]
  n4 = Create User Event(user event datatype=w35) -> (user event=w5:refnum<user-event>)  [unwired: 1 in, 1 out]
  n5 = Bundle By Name(cluster=w39, "talkto event"=w4, "talkback event"=w25) -> (w36:T8)
  n6 = Bundle By Name(cluster=w38, "talkto event"=w5, "talkback event"=w30) -> (w31:T8)
  n7 = Create User Event(user event datatype=w20) -> (user event=w19:refnum<user-event>)  [unwired: 1 in, 1 out]
  n8 = Create User Event(user event datatype=w21) -> (user event=w15:refnum<user-event>)  [unwired: 1 in, 1 out]
  n9 = Create User Event(user event datatype=w27) -> (user event=w26:refnum<user-event>)  [unwired: 1 in, 1 out]
  n10 = Create User Event(user event datatype=w28) -> (user event=w6:refnum<user-event>)  [unwired: 1 in, 1 out]
  n11 = Bundle By Name(cluster=w22, "talkto event"=w15, "talkback event"=w19) -> (w17:T8)
  "pll event pair" <- w17
  n12 = Create User Event(user event datatype=w12) -> (user event=w3:refnum<user-event>)  [unwired: 1 in, 1 out]
  n13 = Create User Event(user event datatype=w11) -> (user event=w9:refnum<user-event>)  [unwired: 1 in, 1 out]
  n14 = Bundle By Name(cluster=w29, "talkto event"=w6, "talkback event"=w26) -> (w18:T8)
  n15 = call "gyro -- launch async sweeper.vi"("sweeper event pair"=w31) -> ("reference out"=→"async sweeper":refnum<vi>, "sweeper event pair OUT"=w24:T8)  [unwired: 9 in]
  "sweeper event pair" <- w24
  n16 = Bundle By Name(cluster=T8 {"talkback event"=refnum, "talkto event"=refnum} ("sweeper pair"), "talkto event"=w3, "talkback event"=w9) -> (w10:T8)
  n17 = call "gyro -- launch async fitter.vi"("fitter pair"=w36) -> ("reference out"=→"async fitter":refnum<vi>, "fitter pair OUT"=w23:T8)  [unwired: 9 in]
  "fitter event pair" <- w23
  n18 = call "gyro -- launch async pll.vi"("pll event pair"=w17) -> ("reference out"=→"pll async reference":refnum<vi>)  [unwired: 10 in]
  n19 = call "gyro -- launch async sourcer.vi"("sourcer pair"=w10) -> ("reference out"=→"async sourcer":refnum<vi>, "fitter pair OUT"=w8:T8)  [unwired: 9 in]
  n20 = call "gyro -- launch async sweeper server.vi"("fitter event pair"=w23, "async sweeper event pair"=w24, "sweeper server event pair"=w18) -> ("reference out"=→"sweeper server reference":refnum<vi>)  [unwired: 8 in]
  n21 = Unbundle By Name(w8) -> ("talkto event"=w7:refnum<user-event>)
  n22 = Create User Event(user event datatype=w42) -> (user event=w2:refnum<user-event>)  [unwired: 1 in, 1 out]
  n23 = register-events(w26, w19, w2) -> (reference out=w44:refnum<event-registration>)  [unwired: 2 in, 1 out]
  n24 = register-events(w2) -> (reference out=w50:refnum<event-registration>)  [unwired: 2 in, 1 out]
  n25 = call "aggregator - vii - real - atomic.vi"("aggregator action"=agregator_--_action."empty!", "requested size"=100, "state IN"=T12 {"requested size"=20, "Array"=[], "actual number of elements"=0}) -> ("state OUT"=w45:T12)  [unwired: 5 in, 3 out]
  n26 = while {
    shift-right: [w53] -> _
    shift-left: w45 -> [w56]
    shift-right: [w54] -> _
    shift-left: w45 -> [w55]
    tunnel: w44 -> [w52]
    tunnel: w7 -> [_]
    stop <- w51 stop-if-true
    n27 = event shown="[0] <pll talkback >: User Event" {
      selector: w52 -> [_ _]
      dyn-events: _ -> [_ _]
      timeout: _ -> [_ _]
      tunnel: w56 -> [w61 w134]
      tunnel: w55 -> [w60 w133]
      tunnel: [w59 w133] -> w54
      tunnel: [w58 w134] -> w53
      tunnel: [_ w131] -> w51
      event User Event {
        n28 = event-data() -> ("message"=w57:enum16{"new", "void"})  [unwired: 1 in]
        n29 = case shown="\"new\"" w57 {
          tunnel: w61 -> [w63 w123]
          tunnel: w60 -> [w62 w120]
          tunnel: [w62 w119] -> w59
          tunnel: [w63 w90] -> w58
          frame "void", Default {
          }
          frame "new" {
            w77 = 0.0 ("new X")
            n30 = call "publish -- pll result.vi"("publisher action"=publisher_action."get") -> ("pll result OUT"=w68:T17)  [unwired: 10 in]
            n31 = local read "plot hist time (sec)"() -> (w84:dbl)
            n32 = Unbundle By Name(w68) -> ("freq (Hz)"=w67:dbl, "gamma (Hz)"=w66:dbl, "Voltage (V)"=w65:cdb)
            "f (Hz)" <- w67
            "G (Hz)" <- w66
            n33 = local read "dt (sec)"() -> (w85:dbl)
            n34 = local read "lorentzian"() -> (w86:T3)
            n35 = control-ref of="Plot: complex plane"() -> (w64:refnum<vi>)
            n36 = Divide(x=w84, y=w85) -> (x/y=w114:dbl)
            n37 = disable-structure shown="Enabled" {
              disable-tunnel: [w128 w130] -> w124
              disable-tunnel: w86 -> [w126 w129]
              disable-tunnel: [w125 w129] -> w88
              frame Disabled {
                n38 = call "lorentzian transformations.vi"("4 corner circle transformation"=four-corner_circle_transformation."get4corners", "lorentzian in"=w126) -> ("lorentzian out"=w125:T3, "4corners our"=w128:T4)  [unwired: 6 in, 2 out]
              }
              frame Enabled {
                n39 = Unbundle By Name(w129) -> ("4corners"=w130:T4)
              }
            }
            n40 = Bundle By Name(cluster=T6 {"freq (Hz)"=0.0, "gamma (Hz)"=0.0, "Voltage (V)"=0.0+0.0i} ("publish message"), "freq (Hz)"=w67, "gamma (Hz)"=w66, "Voltage (V)"=w65) -> (→"publish message":T6)
            n41 = Round To Nearest(number=w114) -> (nearest integer value=w113:dbl)
            n42 = To Long Integer(number=w113) -> (32bit integer=w112:i32)
            n43 = call "aggregator - vii - complex - atomic.vi"("aggregator action"=agregator_--_action."append", "requested size"=w112, "state IN"=w123) -> ("state OUT"=w90:T18)  [unwired: 5 in, 3 out]
            n44 = Complex To Re/Im(x + iy=w65) -> (x=→"zi out Re (V)":dbl, y=→"zi out Im (V)":dbl)
            n45 = call "aggregator - vii - real - atomic.vi"("aggregator action"=agregator_--_action."append", "requested size"=w112, "state IN"=w120) -> ("state OUT"=w119:T12)  [unwired: 5 in, 3 out]
            n46 = call "draw complex lorentzian.vi"("4 corners"=w124) -> ("fancy circles"=→"Plot: complex plane":cluster{dbl[], dbl[]}[])  [unwired: 10 in]
            n47 = Complex To Re/Im(x + iy=w65) -> (x=w81:dbl, y=w82:dbl)
            n48 = call "replace cursor - plot ref - V2.vi"("Plot ref in"=w64, "new X"=w81, "new  Y"=w82, "cursor index"=0, "cursor action"=cursor_action."write", "Color Box"=u32 327424) -> ("Plot ref out"=w83:refnum<vi>)  [unwired: 10 in, 3 out]
            n49 = Unbundle By Name(w119) -> ("Array"=w106:dbl[])
            n50 = Unbundle By Name(w90) -> ("Array"=w107:cdb[])
            n51 = call "replace cursor - plot ref - V2.vi"("Plot ref in"=w83, "new X"=w77, "new  Y"=w77, "cursor index"=1, "cursor action"=cursor_action."write", "Color Box"=u32 5880319) -> ()  [unwired: 10 in, 4 out]
            n52 = call "linear interp iiii- complex - z-omega.vi"("z"=w107, "omega"=w106) -> ("slope"=w105:cdb)  [unwired: 5 in, 8 out]
            n53 = Unbundle By Name(w88) -> ("4corners.z center"=w87:cdb, "A (VHz)"=w100:dbl, "G (Hz)"=w102:dbl)
            n54 = Complex To Polar(r * e^(i*theta)=w105) -> (r=w104:dbl)  [unwired: 1 out]
            n55 = Divide(x=w105, y=w104) -> (x/y=w103:cdb)
            n56 = call "lorentzian transformations.vi"("4 corner circle transformation"=four-corner_circle_transformation."get4corners", "lorentzian in"="lorentzian -- hist") -> ("4corners our"=w111:T4)  [unwired: 6 in, 3 out]
            n57 = Reciprocal(x=w102) -> (1/x=w101:dbl)
            n58 = Complex To Re/Im(x + iy=w107) -> (x=w117:dbl[], y=w116:dbl[])
            n59 = Compound Arithmetic op=MULTIPLY(w103, w101, w100, 1.1 ("value")) -> (w93:cdb)
            n60 = call "draw complex lorentzian.vi"("4 corners"=w111) -> ("fancy circles"=w109:cluster{dbl[], dbl[]}[])  [unwired: 10 in]
            n61 = Bundle(w117, w116) -> (w118:cluster{dbl[], dbl[]})  [unwired: 1 in]
            n62 = Add(x=w87, y=w93) -> (x+y=w99:cdb)
            n63 = Subtract(x=w87, y=w93) -> (x-y=w98:cdb)
            n64 = Complex To Re/Im(x + iy=w99) -> (x=w97:dbl, y=w95:dbl)
            n65 = Complex To Re/Im(x + iy=w98) -> (x=w96:dbl, y=w94:dbl)
            n66 = call "draw a line.vi"("y1"=w94, "y0"=w95, "x1"=w96, "x0"=w97) -> ("output cluster"=w91:cluster{dbl[], dbl[]})  [unwired: 7 in]
            n67 = Build Array (concatenate)(w118, w109, w91) -> (→"Plot: complex- hist":cluster{dbl[], dbl[]}[])
          }
        }
      }
      event User Event {
        n68 = event-data() -> ("pll internal user event action"=w132:T11)  [unwired: 1 in]
        n69 = case shown="\"exit\"" w132 {
          tunnel: [_ TRUE] -> w131
          frame "void", Default {
          }
          frame "exit" {
          }
        }
      }
    }
  }
  n70 = control-ref of="Plot: complex- hist"() -> (w46:refnum<vi>)
  n71 = control-ref of="Plot: complex plane"() -> (w43:refnum<vi>)
  n72 = while {
    tunnel: w50 -> [w145]
    tunnel: w2 -> [w144]
    tunnel: w43 -> [w143]
    tunnel: w46 -> [w142]
    tunnel: w15 -> [w141]
    tunnel: w18 -> [_]
    tunnel: w6 -> [w140]
    tunnel: w5 -> [w139]
    tunnel: w4 -> [w138]
    tunnel: w3 -> [w137]
    stop <- w136 stop-if-true
    n73 = event shown="[13] Key Down" {
      selector: w145 -> [_ _ _ _ _ _ _ _ _ _ _ _ _ _]
      dyn-events: _ -> [_ _ _ _ _ _ _ _ _ _ _ _ _ _]
      timeout: _ -> [_ _ _ _ _ _ _ _ _ _ _ _ _ _]
      tunnel: [_ "(*) pll" "(*) sourcer" "(*) fitter" "(*) sweeper" "(*) sweeper server" "exit!" "toggle PLL! :@" _ "reset freq! :r" "reset lor! :q" "reset lorentzian from basic" "save lor for later" _] -> _
      tunnel: w144 -> [w152 w240 w243 w246 w249 w252 w254 w258 _ w293 w296 _ _ w307]
      tunnel: w143 -> [w153 _ _ _ _ _ _ _ w264 _ _ _ _ w306]
      tunnel: w142 -> [_ _ _ _ _ _ _ _ _ _ _ _ _ w305]
      tunnel: w141 -> [w151 _ _ _ _ _ _ _ _ _ _ _ _ _]
      tunnel: w140 -> [w150 _ _ _ _ _ _ _ _ _ _ _ _ _]
      tunnel: w139 -> [w149 _ _ _ _ _ _ _ _ _ _ _ _ _]
      tunnel: w138 -> [w148 _ _ _ _ _ _ _ _ _ _ _ _ _]
      tunnel: w137 -> [w147 _ _ _ _ _ _ _ _ _ _ _ _ _]
      tunnel: [w146 _ _ _ _ _ _ _ _ _ _ _ _ _] -> w136
      event User Event {
        n74 = event-data() -> ("pll internal user event action"=w154:T11)  [unwired: 1 in]
        n75 = case shown="\"exit\"" w154 {
          tunnel: w153 -> [_ _ _ _ _ _ _ _ _ _ _ _ _ w232 _]
          tunnel: w152 -> [_ _ w159 _ _ _ w175 _ _ _ _ _ w216 _ w234]
          tunnel: w151 -> [_ w156 w164 w167 w170 w171 w182 _ _ _ _ _ _ _ _]
          tunnel: w150 -> [_ _ _ _ _ _ w181 _ _ _ _ _ _ _ _]
          tunnel: w149 -> [_ _ _ _ _ _ w180 _ _ _ _ _ _ _ _]
          tunnel: w148 -> [_ _ _ _ _ _ w179 _ _ _ _ _ _ _ _]
          tunnel: w147 -> [_ _ _ _ _ _ w178 _ _ _ _ _ _ _ _]
          tunnel: [_ _ _ _ _ _ TRUE _ _ _ _ _ _ _ _] -> w146
          frame "void", Default {
          }
          frame "accept frequency" {
            n76 = Generate User Event(user event=w156, event data cluster=T10 {"message"=enum."reset"} ("event data")) -> ()  [unwired: 2 in, 2 out]
          }
          frame "accept lorentzian" {
            n77 = Generate User Event(user event=w159, event data cluster=pll_internal_user_event_action."update cursors" ("event data")) -> ()  [unwired: 2 in, 2 out]
            n78 = call "publish -- lorentzian.vi"("publisher action"=publisher_action."get") -> ("lorentzian OUT"=w163:T3)  [unwired: 10 in]
            n79 = Generate User Event(user event=w164, event data cluster=T10 {"message"=enum."update request"} ("event data")) -> ()  [unwired: 2 in, 2 out]
            n80 = call "lorentzian transformations.vi"("4 corner circle transformation"=four-corner_circle_transformation."get4corners", "lorentzian in"=w163) -> ("lorentzian out"=w162:T3)  [unwired: 6 in, 3 out]
            n81 = local write "lorentzian -- hist"(w162) -> ()
            n82 = local write "lorentzian"(w162) -> ()
          }
          frame "pause pll" {
            n83 = Generate User Event(user event=w167, event data cluster=T10 {"message"=enum."pause"} ("event data")) -> ()  [unwired: 2 in, 2 out]
            n84 = local write "PLL is ON"(FALSE ("PLL ON")) -> ()
          }
          frame "unpause pll" {
            n85 = Generate User Event(user event=w170, event data cluster=T10 {"message"=enum."unpause"} ("event data")) -> ()  [unwired: 2 in, 2 out]
            n86 = local write "PLL is ON"(TRUE ("PLL ON")) -> ()
          }
          frame "start pll async" {
            n87 = Generate User Event(user event=w171, event data cluster=T10 {"message"=enum."start"} ("event data")) -> ()  [unwired: 2 in, 2 out]
          }
          frame "exit" {
            w177 = T10 {"message"=enum."exit"} ("event data")
            n88 = Generate User Event(user event=w175, event data cluster=pll_internal_user_event_action."exit" ("event data")) -> ()  [unwired: 2 in, 2 out]
            n89 = Generate User Event(user event=w182, event data cluster=w177) -> ()  [unwired: 2 in, 2 out]
            n90 = Generate User Event(user event=w179, event data cluster=w177) -> ()  [unwired: 2 in, 2 out]
            n91 = Generate User Event(user event=w178, event data cluster=w177) -> ()  [unwired: 2 in, 2 out]
            n92 = Generate User Event(user event=w180, event data cluster=w177) -> ()  [unwired: 2 in, 2 out]
            n93 = Generate User Event(user event=w181, event data cluster=w177) -> ()  [unwired: 2 in, 2 out]
            n94 = local write "PLL is ON"(FALSE ("PLL ON")) -> ()
            n95 = local write "Stoped?"(TRUE ("Stoped?")) -> ()
          }
          frame "gear pll async" {
            n96 = local read "pll async reference"() -> (w185:refnum<vi>)
            n97 = property class="VI Interface Type 0"(reference=w185) -> ("FP.State"=w184:T19)  [unwired: 1 in, 2 out]
            n98 = case shown="\"Standard\", Default" w184 {
              tunnel: w185 -> [w188 w189]
              frame "Closed" {
                n99 = invoke class="VI Interface Type 0" method="FP.Open"(reference=w188, "Activate"=TRUE ("Activate?"), "State"=T19."Standard" ("Front Panel Window:State")) -> ()  [unwired: 2 in, 5 out]
              }
              frame "Standard", Default {
                n100 = invoke class="VI Interface Type 0" method="FP.Close"(reference=w189) -> ()  [unwired: 2 in, 3 out]
              }
            }
          }
          frame "gear server sweeper" {
            n101 = local read "sweeper server reference"() -> (w191:refnum<vi>)
            n102 = property class="VI Interface Type 1"(reference=w191) -> ("FP.State"=w190:T19)  [unwired: 1 in, 2 out]
            n103 = case shown="\"Standard\", Default" w190 {
              tunnel: w191 -> [w194 w195]
              frame "Closed" {
                n104 = invoke class="VI Interface Type 1" method="FP.Open"(reference=w194, "Activate"=TRUE ("Activate?"), "State"=T19."Standard" ("Front Panel Window:State")) -> ()  [unwired: 2 in, 5 out]
              }
              frame "Standard", Default {
                n105 = invoke class="VI Interface Type 1" method="FP.Close"(reference=w195) -> ()  [unwired: 2 in, 3 out]
              }
            }
          }
          frame "gear sweeper async" {
            n106 = local read "async sweeper"() -> (w197:refnum<vi>)
            n107 = property class="VI Interface Type 0"(reference=w197) -> ("FP.State"=w196:T19)  [unwired: 1 in, 2 out]
            n108 = case shown="\"Standard\", Default" w196 {
              tunnel: w197 -> [w200 w201]
              frame "Closed" {
                n109 = invoke class="VI Interface Type 0" method="FP.Open"(reference=w200, "Activate"=TRUE ("Activate?"), "State"=T19."Standard" ("Front Panel Window:State")) -> ()  [unwired: 2 in, 5 out]
              }
              frame "Standard", Default {
                n110 = invoke class="VI Interface Type 0" method="FP.Close"(reference=w201) -> ()  [unwired: 2 in, 3 out]
              }
            }
          }
          frame "gear fitter" {
            n111 = local read "async fitter"() -> (w203:refnum<vi>)
            n112 = property class="VI Interface Type 0"(reference=w203) -> ("FP.State"=w202:T19)  [unwired: 1 in, 2 out]
            n113 = case shown="\"Standard\", Default" w202 {
              tunnel: w203 -> [w206 w207]
              frame "Closed" {
                n114 = invoke class="VI Interface Type 0" method="FP.Open"(reference=w206, "Activate"=TRUE ("Activate?"), "State"=T19."Standard" ("Front Panel Window:State")) -> ()  [unwired: 2 in, 5 out]
              }
              frame "Standard", Default {
                n115 = invoke class="VI Interface Type 0" method="FP.Close"(reference=w207) -> ()  [unwired: 2 in, 3 out]
              }
            }
          }
          frame "gear sourcer" {
            n116 = local read "async sourcer"() -> (w209:refnum<vi>)
            n117 = property class="VI Interface Type 0"(reference=w209) -> ("FP.State"=w208:T19)  [unwired: 1 in, 2 out]
            n118 = case shown="\"Standard\", Default" w208 {
              tunnel: w209 -> [w212 w213]
              frame "Closed" {
                n119 = invoke class="VI Interface Type 0" method="FP.Open"(reference=w212, "Activate"=TRUE ("Activate?"), "State"=T19."Standard" ("Front Panel Window:State")) -> ()  [unwired: 2 in, 5 out]
              }
              frame "Standard", Default {
                n120 = invoke class="VI Interface Type 0" method="FP.Close"(reference=w213) -> ()  [unwired: 2 in, 3 out]
              }
            }
          }
          frame "toggle pll async" {
            n121 = local read "PLL is ON"() -> (w215:bool)
            n122 = case shown="False" w215 {
              tunnel: [pll_internal_user_event_action."unpause pll" ("event data") pll_internal_user_event_action."pause pll" ("event data")] -> w214
              frame False {
              }
              frame True {
              }
            }
            n123 = Generate User Event(user event=w216, event data cluster=w214) -> ()  [unwired: 2 in, 2 out]
          }
          frame "update cursors" {
            n124 = local read "lorentzian"() -> (w219:T3)
            n125 = Unbundle By Name(w219) -> ("4corners.z(inf)"=w227:cdb, "4corners.z(0)"=w220:cdb)
            n126 = Complex To Re/Im(x + iy=w227) -> (x=w229:dbl, y=w228:dbl)
            n127 = Complex To Re/Im(x + iy=w220) -> (x=w223:dbl, y=w222:dbl)
            n128 = call "replace cursor - plot ref - V2.vi"("Plot ref in"=w232, "new X"=w229, "new  Y"=w228, "cursor index"=2, "cursor action"=cursor_action."write", "Color Box"=u32 16746738) -> ()  [unwired: 10 in, 4 out]
            n129 = call "replace cursor - plot ref - V2.vi"("Plot ref in"=w232, "new X"=w223, "new  Y"=w222, "cursor index"=3, "cursor action"=cursor_action."write", "Color Box"=u32 10682154) -> ()  [unwired: 10 in, 4 out]
          }
          frame "toggle sweeper" {
            n130 = case shown="True" "PLL is ON" {
              tunnel: w234 -> [_ w236]
              frame False {
              }
              frame True {
                n131 = Generate User Event(user event=w236, event data cluster=pll_internal_user_event_action."pause pll" ("event data")) -> ()  [unwired: 2 in, 2 out]
              }
            }
            n132 = Generate User Event(user event=w234, event data cluster=pll_internal_user_event_action."start sweeper" ("event data")) -> ()  [unwired: 2 in, 2 out]
          }
        }
      }
      event "(*) pll": Value Change {
        n133 = event-data() -> ()  [unwired: 1 in, 6 out]
        n134 = Generate User Event(user event=w240, event data cluster=pll_internal_user_event_action."gear pll async" ("event data")) -> ()  [unwired: 2 in, 2 out]
      }
      event "(*) sourcer": Value Change {
        n135 = event-data() -> ()  [unwired: 1 in, 6 out]
        n136 = Generate User Event(user event=w243, event data cluster=pll_internal_user_event_action."gear sourcer" ("event data")) -> ()  [unwired: 2 in, 2 out]
      }
      event "(*) fitter": Value Change {
        n137 = event-data() -> ()  [unwired: 1 in, 6 out]
        n138 = Generate User Event(user event=w246, event data cluster=pll_internal_user_event_action."gear fitter" ("event data")) -> ()  [unwired: 2 in, 2 out]
      }
      event "(*) sweeper": Value Change {
        n139 = event-data() -> ()  [unwired: 1 in, 6 out]
        n140 = Generate User Event(user event=w249, event data cluster=pll_internal_user_event_action."gear sweeper async" ("event data")) -> ()  [unwired: 2 in, 2 out]
      }
      event "(*) sweeper server": Value Change {
        n141 = event-data() -> ()  [unwired: 1 in, 6 out]
        n142 = Generate User Event(user event=w252, event data cluster=pll_internal_user_event_action."gear server sweeper" ("event data")) -> ()  [unwired: 2 in, 2 out]
      }
      event "exit!": Value Change {
        n143 = event-data() -> ()  [unwired: 1 in, 6 out]
        n144 = Generate User Event(user event=w254, event data cluster=pll_internal_user_event_action."exit" ("event data")) -> ()  [unwired: 2 in, 2 out]
      }
      event "toggle PLL! :@": Value Change {
        n145 = event-data() -> ()  [unwired: 1 in, 1 out]
        n146 = Generate User Event(user event=w258, event data cluster=pll_internal_user_event_action."toggle pll async" ("event data")) -> ()  [unwired: 2 in, 2 out]
      }
      event "Plot: complex plane": Cursor Move {
        n147 = event-data() -> ("CursIdx"=w263:i32)  [unwired: 1 in]
        n148 = local read "lorentzian"() -> (w262:T3)
        n149 = case shown="2" w263 {
          selector: w263 -> [_ w276 w286]
          tunnel: w264 -> [_ w270 w285]
          tunnel: w262 -> [w265 w266 w284]
          tunnel: [w265 w267 w281] -> w260
          frame 0, Default {
          }
          frame 2 {
            n150 = call "replace cursor - plot ref - V2.vi"("Plot ref in"=w270, "cursor index"=w276, "cursor action"=cursor_action."read") -> ("read X"=w278:dbl, "read Y"=w279:dbl)  [unwired: 13 in, 2 out]
            n151 = Re/Im To Complex(1:w279, 2:w278) -> (0:w277:cdb)
            n152 = Bundle By Name(cluster=w266, "bg (V)"=w277) -> (w275:T3)
            n153 = call "lorentzian transformations.vi"("4 corner circle transformation"=four-corner_circle_transformation."get4corners", "lorentzian in"=w275) -> ("lorentzian out"=w267:T3)  [unwired: 6 in, 3 out]
            n154 = Unbundle By Name(w267) -> ("4corners.z(0)"=w273:cdb)
            n155 = Complex To Re/Im(x + iy=w273) -> (x=w272:dbl, y=w271:dbl)
            n156 = call "replace cursor - plot ref - V2.vi"("Plot ref in"=w270, "new X"=w272, "new  Y"=w271, "cursor index"=3, "cursor action"=cursor_action."write") -> ()  [unwired: 11 in, 4 out]
          }
          frame 3 {
            n157 = call "replace cursor - plot ref - V2.vi"("Plot ref in"=w285, "cursor index"=w286, "cursor action"=cursor_action."read") -> ("read X"=w288:dbl, "read Y"=w289:dbl)  [unwired: 13 in, 2 out]
            n158 = Re/Im To Complex(1:w289, 2:w288) -> (0:w287:cdb)
            n159 = Bundle By Name(cluster=w284, "4corners.z(0)"=w287) -> (w283:T3)
            n160 = call "lorentzian transformations.vi"("4 corner circle transformation"=four-corner_circle_transformation."update lorentzian -- from z0", "lorentzian in"=w283) -> ("lorentzian out"=w281:T3)  [unwired: 6 in, 3 out]
          }
        }
        n161 = call "lorentzian transformations.vi"("4 corner circle transformation"=four-corner_circle_transformation."get4corners", "lorentzian in"=w260) -> ("lorentzian out"=w259:T3)  [unwired: 6 in, 3 out]
        n162 = local write "lorentzian"(w259) -> ()
      }
      event "reset freq! :r": Value Change {
        n163 = event-data() -> ()  [unwired: 1 in, 6 out]
        n164 = Generate User Event(user event=w293, event data cluster=pll_internal_user_event_action."accept frequency" ("event data")) -> ()  [unwired: 2 in, 2 out]
      }
      event "reset lor! :q": Value Change {
        n165 = event-data() -> ()  [unwired: 1 in, 6 out]
        n166 = Generate User Event(user event=w296, event data cluster=pll_internal_user_event_action."accept lorentzian" ("event data")) -> ()  [unwired: 2 in, 2 out]
      }
      event "reset lorentzian from basic": Value Change {
        n167 = event-data() -> ()  [unwired: 1 in, 6 out]
        n168 = local read "lorentzian -- basic"() -> (w298:T3)
        n169 = call "lorentzian transformations.vi"("4 corner circle transformation"=four-corner_circle_transformation."get4corners", "lorentzian in"=w298) -> ("lorentzian out"=w297:T3)  [unwired: 6 in, 3 out]
        n170 = local write "lorentzian"(w297) -> ()
      }
      event "save lor for later": Value Change {
        n171 = event-data() -> ()  [unwired: 1 in, 6 out]
        n172 = local read "lorentzian"() -> (w302:T3)
        n173 = call "lorentzian transformations.vi"("4 corner circle transformation"=four-corner_circle_transformation."get4corners", "lorentzian in"=w302) -> ("lorentzian out"=w301:T3)  [unwired: 6 in, 3 out]
        n174 = local write "lorentzian -- basic"(w301) -> ()
      }
      event Key Down {
        n175 = event-data() -> ("Char"=w309:i16, "VKey"=w311:T5)  [unwired: 1 in]
        "Char" <- w309
        "VKey" <- w311
        n176 = Build Array(w309) -> (w310:i16[])
        n177 = Byte Array To String(unsigned byte array=w310) -> (string=w308:string)
        n178 = case shown="\"ASCII\", Default" w311 {
          selector: w311 -> [_ _ _ _ w394]
          tunnel: w309 -> [_ _ _ _ _]
          tunnel: w308 -> [w315 _ _ _ _]
          tunnel: w307 -> [w314 _ _ _ _]
          tunnel: w306 -> [w313 _ _ _ w393]
          tunnel: w305 -> [w312 _ _ _ w392]
          frame "ASCII", Default {
            n179 = case shown="\"q\"" w315 {
              selector: w315 -> [_ w318 _ w328 _ _ _]
              tunnel: w314 -> [_ _ w326 _ w386 w388 w390]
              tunnel: w313 -> [_ w317 _ _ _ _ _]
              tunnel: w312 -> [_ w316 _ _ _ _ _]
              frame "0", Default {
              }
              frame "<", ">", "?", "A", "z" {
                n180 = case shown="\"A\"" w318 {
                  tunnel: [cursor_action."zoom out 20%" ("cursor action") cursor_action."zoom in 20%" ("cursor action") cursor_action."smart zoom out&aspect" ("cursor action") cursor_action."smart zoom out" ("cursor action") cursor_action."zoom to aspect ratio 1" ("cursor action")] -> w319
                  frame ">" {
                  }
                  frame "<" {
                  }
                  frame "?" {
                  }
                  frame "A" {
                  }
                  frame "z", Default {
                  }
                }
                n181 = call "replace cursor - plot ref - V2.vi"("Plot ref in"=w317, "cursor action"=w319) -> ()  [unwired: 14 in, 4 out]
                n182 = call "replace cursor - plot ref - V2.vi"("Plot ref in"=w316, "cursor action"=w319) -> ()  [unwired: 14 in, 4 out]
              }
              frame "r" {
                (unwired) "reset frequency" ("event data")
                n183 = Generate User Event(user event=w326, event data cluster=pll_internal_user_event_action."accept frequency" ("event data")) -> ()  [unwired: 2 in, 2 out]
              }
              frame "'", ";", "[", "]", "{", "}" {
                n184 = control-ref of="PID parameters :{}[];'"() -> (w327:refnum<vi>)
                n185 = case shown="\"]\"" w328 {
                  tunnel: w327 -> [w333 w342 w351 w360 w369 w379]
                  frame "[" {
                    n186 = property class="Clust (strict)"(reference=w333) -> (reference out=w332:refnum<vi>, "Value"=w331:T2)  [unwired: 1 in, 1 out]
                    n187 = in-place {
                      in-place-border: 0.9 -> [w336]
                      n188 = in-place-cluster #1(w331) -> ("P (sec)"=w334:dbl, "I (sec)"=w337:dbl)
                      n189 = Multiply(x=w337, y=w336) -> (x*y=w335:dbl)
                      n190 = in-place-cluster #1("P (sec)"=w334, "I (sec)"=w335) -> (w330:T2)
                    }
                    n191 = property class="Clust (strict)"(reference=w332, "Value"=w330) -> ()  [unwired: 1 in, 2 out]
                  }
                  frame "]" {
                    n192 = property class="Clust (strict)"(reference=w342) -> (reference out=w341:refnum<vi>, "Value"=w340:T2)  [unwired: 1 in, 1 out]
                    n193 = in-place {
                      in-place-border: 1.1 -> [w345]
                      n194 = in-place-cluster #2(w340) -> ("P (sec)"=w343:dbl, "I (sec)"=w346:dbl)
                      n195 = Multiply(x=w346, y=w345) -> (x*y=w344:dbl)
                      n196 = in-place-cluster #2("P (sec)"=w343, "I (sec)"=w344) -> (w339:T2)
                    }
                    n197 = property class="Clust (strict)"(reference=w341, "Value"=w339) -> ()  [unwired: 1 in, 2 out]
                  }
                  frame "}" {
                    n198 = property class="Clust (strict)"(reference=w351) -> (reference out=w350:refnum<vi>, "Value"=w349:T2)  [unwired: 1 in, 1 out]
                    n199 = in-place {
                      in-place-border: 1.1 -> [w355]
                      n200 = in-place-cluster #3(w349) -> ("P (sec)"=w354:dbl, "I (sec)"=w352:dbl)
                      n201 = Multiply(x=w354, y=w355) -> (x*y=w353:dbl)
                      n202 = in-place-cluster #3("P (sec)"=w353, "I (sec)"=w352) -> (w348:T2)
                    }
                    n203 = property class="Clust (strict)"(reference=w350, "Value"=w348) -> ()  [unwired: 1 in, 2 out]
                  }
                  frame "{", Default {
                    n204 = property class="Clust (strict)"(reference=w360) -> (reference out=w359:refnum<vi>, "Value"=w358:T2)  [unwired: 1 in, 1 out]
                    n205 = in-place {
                      in-place-border: 0.9 -> [w364]
                      n206 = in-place-cluster #4(w358) -> ("P (sec)"=w363:dbl, "I (sec)"=w361:dbl)
                      n207 = Multiply(x=w363, y=w364) -> (x*y=w362:dbl)
                      n208 = in-place-cluster #4("P (sec)"=w362, "I (sec)"=w361) -> (w357:T2)
                    }
                    n209 = property class="Clust (strict)"(reference=w359, "Value"=w357) -> ()  [unwired: 1 in, 2 out]
                  }
                  frame "'" {
                    n210 = property class="Clust (strict)"(reference=w369) -> (reference out=w368:refnum<vi>, "Value"=w367:T2)  [unwired: 1 in, 1 out]
                    n211 = in-place {
                      in-place-border: 1.1 -> [w370]
                      n212 = in-place-cluster #5(w367) -> ("P (sec)"=w374:dbl, "I (sec)"=w372:dbl)
                      n213 = Multiply(x=w374, y=w370) -> (x*y=w373:dbl)
                      n214 = Multiply(x=w372, y=w370) -> (x*y=w371:dbl)
                      n215 = in-place-cluster #5("P (sec)"=w373, "I (sec)"=w371) -> (w366:T2)
                    }
                    n216 = property class="Clust (strict)"(reference=w368, "Value"=w366) -> ()  [unwired: 1 in, 2 out]
                  }
                  frame ";" {
                    n217 = property class="Clust (strict)"(reference=w379) -> (reference out=w378:refnum<vi>, "Value"=w377:T2)  [unwired: 1 in, 1 out]
                    n218 = in-place {
                      in-place-border: 0.9 -> [w380]
                      n219 = in-place-cluster #6(w377) -> ("P (sec)"=w384:dbl, "I (sec)"=w382:dbl)
                      n220 = Multiply(x=w384, y=w380) -> (x*y=w383:dbl)
                      n221 = Multiply(x=w382, y=w380) -> (x*y=w381:dbl)
                      n222 = in-place-cluster #6("P (sec)"=w383, "I (sec)"=w381) -> (w376:T2)
                    }
                    n223 = property class="Clust (strict)"(reference=w378, "Value"=w376) -> ()  [unwired: 1 in, 2 out]
                  }
                }
              }
              frame "@" {
                (unwired) "toggle PLL" ("event data")
                n224 = Generate User Event(user event=w386, event data cluster=pll_internal_user_event_action."toggle pll async" ("event data")) -> ()  [unwired: 2 in, 2 out]
              }
              frame "#" {
                (unwired) "(sweeper) sweep!" ("event data")
                n225 = Generate User Event(user event=w388, event data cluster=pll_internal_user_event_action."toggle sweeper" ("event data")) -> ()  [unwired: 2 in, 2 out]
              }
              frame "q" {
                (unwired) "reset lorentzian" ("event data")
                n226 = Generate User Event(user event=w390, event data cluster=pll_internal_user_event_action."accept lorentzian" ("event data")) -> ()  [unwired: 2 in, 2 out]
              }
            }
          }
          frame "Escape" {
          }
          frame "PageUp" {
          }
          frame "PageDown" {
          }
          frame "Up".."Right" {
            n227 = case shown="\"Down\"" w394 {
              tunnel: [cursor_action."move range right 20%" ("cursor action") cursor_action."move range left 20%" ("cursor action") cursor_action."move range up 20%" ("cursor action") cursor_action."move range down 20%" ("cursor action")] -> w391
              frame "Right", Default {
              }
              frame "Left" {
              }
              frame "Up" {
              }
              frame "Down" {
              }
            }
            n228 = call "replace cursor - plot ref - V2.vi"("Plot ref in"=w393, "cursor action"=w391) -> ()  [unwired: 14 in, 4 out]
            n229 = call "replace cursor - plot ref - V2.vi"("Plot ref in"=w392, "cursor action"=w391) -> ()  [unwired: 14 in, 4 out]
          }
        }
      }
    }
  }
  n230 = while {
    stop <- w399 stop-if-true
    n231 = local read "publish message"() -> (w403:T6)
    n232 = Unbundle By Name(w403) -> ("freq (Hz)"=w402:dbl, "Voltage (V)"=w401:cdb, "gamma (Hz)"=w400:dbl)
    n233 = Wait (ms)(milliseconds to wait=u32 10) -> ()  [unwired: 1 out]
    n234 = local read "Stoped?"() -> (w399:bool)
    n235 = call "publish -- get frequency and voltage.vi"("publisher action"=publisher_action."set", "gamma IN (Hz)"=w400, "Voltage IN (V)"=w401, "freq IN (Hz)"=w402) -> ()  [unwired: 5 in, 3 out]
  }
  "Stoped?" <- FALSE ("Stoped?")
